vi "Configure Limit Test Settings.vi"(6 "Component Binning Mode (0:Immediate)":u16(ring) items=["Immediate", "After Final Test"], 8 "error in (no error)":errorcluster, 9 "Test I/O Mode (0:Grading)":u16(ring) items=["Grading", "Sorting"], 10 "Test Value Source  (0: Voltage)":u16(ring) items=["Voltage", "Current", "Resistance"], 11 "VISA resource name":refnum<visa-resource-name>) -> (0 "error out":errorcluster, 3 "VISA resource name out":refnum<visa-resource-name>)   [LabVIEW 2018, in "Keithley 24XX.lvlib"]
doc: "Configures limit testing settings, such as the source of the tested value, binning, and I/O settings."
uses:
  Keithley 24XX.lvlib
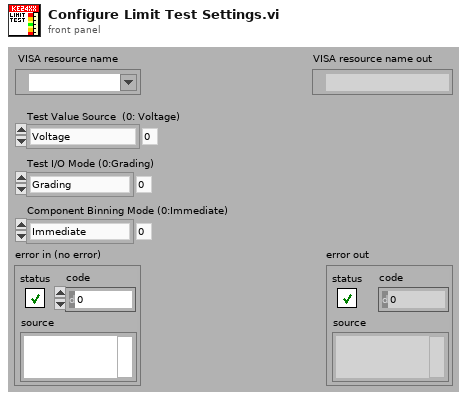
[diagram p1: front panel]
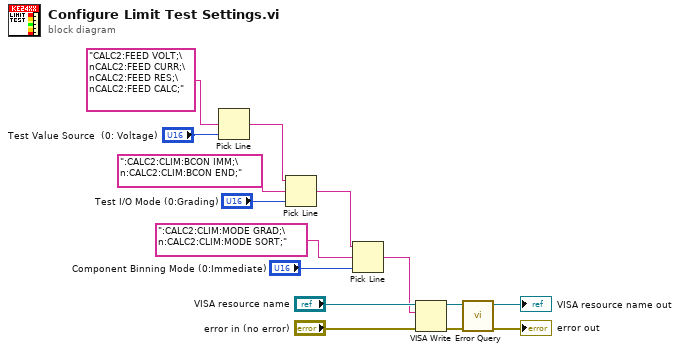
[diagram p0: block diagram]
diagram:
  n1 = Pick Line(multi-line string="CALC2:FEED VOLT;\nCALC2:FEED CURR;\nCALC2:FEED RES;\nCALC2:FEED CALC;", line index="Test Value Source  (0: Voltage)") -> (output string=w3:string)  [unwired: 1 in]
  n2 = Pick Line(string ("")=w3, multi-line string=":CALC2:CLIM:BCON IMM;\n:CALC2:CLIM:BCON END;", line index="Test I/O Mode (0:Grading)") -> (output string=w2:string)
  n3 = Pick Line(string ("")=w2, multi-line string=":CALC2:CLIM:MODE GRAD;\n:CALC2:CLIM:MODE SORT;", line index="Component Binning Mode (0:Immediate)") -> (output string=w1:string)
  n4 = VISA Write(VISA resource name="VISA resource name", write buffer=w1, error in (no error)="error in (no error)") -> (VISA resource name out=w11:refnum<visa-resource-name>, error out=w10:errorcluster)  [unwired: 1 out]
  n5 = call "Error Query.vi"("error in (no error)"=w10, "VISA resource name"=w11) -> ("error out"=→"error out":errorcluster, "VISA resource name out"=→"VISA resource name out":refnum<visa-resource-name>)  [unwired: 6 in, 2 out]
